vi "setCaption&LabelVisibility.vi"(8 "error in (no error)":errorcluster, 9 "Label.Visible":bool, 10 "Caption.Visible":bool, 11 "Control in":refnum<vi>) -> (0 "error out":errorcluster, 3 "Control out":refnum<vi>)   [LabVIEW 2023]
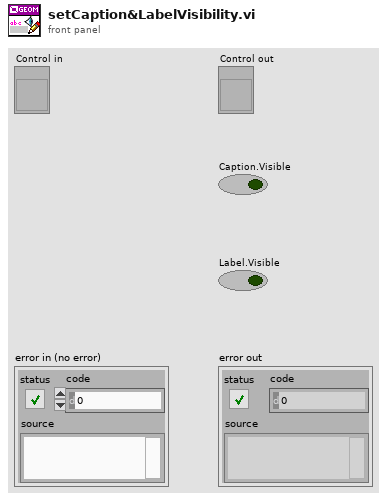
[diagram p1: front panel]
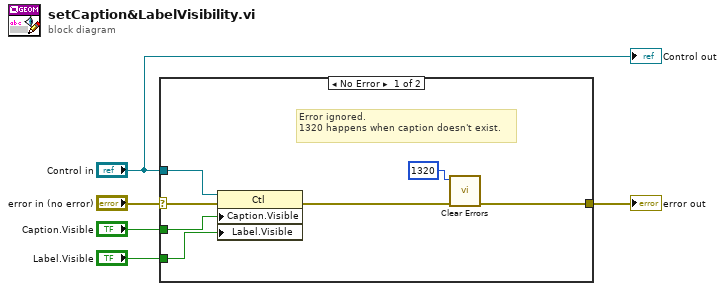
[diagram p0: block diagram]
diagram:
  n1 = case shown="No Error" "error in (no error)" {
    selector: "error in (no error)" -> [w12 w13]
    tunnel: [w6 w13] -> w4
    tunnel: "Caption.Visible" -> [w11 _]
    tunnel: "Label.Visible" -> [w10 _]
    tunnel: "Control in" -> [w9 _]
    frame No Error {
      # "Error ignored.\n1320 happens when caption doesn't exist."
      n2 = property class="Ctl"(reference=w9, error in=w12, "Caption.Visible"=w11, "Label.Visible"=w10) -> (error out=w7:errorcluster)  [unwired: 1 out]
      n3 = call <vilib>:"Clear Errors.vi"("error in (no error)"=w7, "specific error code to clear (0: all)"=1320) -> ("error out"=w6:errorcluster)  [unwired: 4 in, 1 out]
    }
    frame Error {
    }
  }
  "error out" <- w4
  "Control out" <- "Control in"
